vi "COD主界面（列队使用）.vi"() -> (8 "多列列表框":i32(listbox))   [LabVIEW 2016, in "斯坦道CODMn.lvlib"]
uses:
  <vilib>/Utility/miscctls.llb/LVPointTypeDef.ctl
  <vilib>/ptbypt/NI_PtbyPt.lvlib
panel:
  in  "温度补偿":bool
  in  "周期设置":bool
  out "F5":dbl
  out "F4":dbl
  out "F3":dbl
  out "F2":dbl
  out "F1":dbl
  out "F0":dbl
  out "消解压力kPa":dbl format="%#.2f"
  out "权限等级":string
  in  "布尔":bool
  in  "查看曲线":bool
  out "氢氧化钠":dbl
  in  "序列号变更":bool
  out "模块版本号":string
  in  "更新程序":bool
  out "进样无液体告警":bool
  out "60分钟超时报警":bool
  in  "仪器参数":bool
  in  "释放串口":bool
  in  "打开串口":bool
  out "报警数字":i16
  out "CODMn工作状态":T1(ring)
  out "ORP-K":string
  out "ORP-B":string
  out "ORP-A":string
  out "基本量程(显示)":string
  out "测量模式(显示)":string
  out "数据时间":string
  out "断电排液标记":bool
  out "COM":string
  out "空白测试标记":bool
  out "跨度核查标记":bool
  in  "手动控制":bool
  out "启动时间":timestamp format="%<%Y/%m/%d %H:%M:%S>T"
  out "零点核查标记":bool
  out "排液故障":bool
  out "进水样超量程":bool
  out "标样核查标记":bool
  out "平行样测量":bool
  out "加标回收测量":bool
  out "质控样测量":bool
  out "待机":bool
  out "校标错误":bool
  out "校零错误":bool
  out "测量错误":bool
  out "草酸钠报警":bool
  out "高锰酸钾报警":bool
  out "加热故障":bool
  out "温控器故障":bool
  out "ORP故障":bool
  out "排液标记":bool
  out "故障标记":bool
  out "校标标记":bool
  out "校零标记":bool
  out "通讯状态":bool
  out "水样测量":bool
  in  "返回":bool
  in  "校准配置":bool
  out "标度滴定值":dbl
  out "零点滴定值":dbl
  in  "保存":bool
  in  "关闭":bool
  out "仪器时间":timestamp format="%<%Y/%m/%d %H:%M:%S>T"
  out "秒":u16
  out "分":u16
  out "COD浓度（mg/L)":dbl format="%.2g"
  out "进样管":dbl
  out "高锰酸钾":dbl
  out "草酸钠":dbl
  out "硫酸":dbl
  out "实时ORP/光值":dbl
  out "消解温度℃":dbl
  out "加热":bool
  out "搅拌":bool
  out "进硫酸":bool
  out "进加标回收样":bool
  out "进零点核查样":bool
  out "进标液":bool
  out "进蒸馏水":bool
  out "进水样":bool
  out "进草酸钠":bool
  out "进高锰酸钾":bool
  in  "启动":bool
  in  "故障清除":bool
  in  "参数配置":bool
  in  "停止":bool
  in  "单步启动":bool
  out "系统时间":timestamp
  in  "时间校准":bool
  out "模式（受控）":u16
  # "测试时长："
  # "注：遇到加热故障和排液故障时仪器不能正常启动，\n必须排查故障并点击报警清除按钮方可运行。"
  # "mg/L"
  # "校零校标结果"
  # "校零结果："
  # "校零滴定值："
  # "校标结果："
  # "标度滴定值："
  # "零点泵计量值："
  # "标度泵计量值："
  # "校准配置界面"
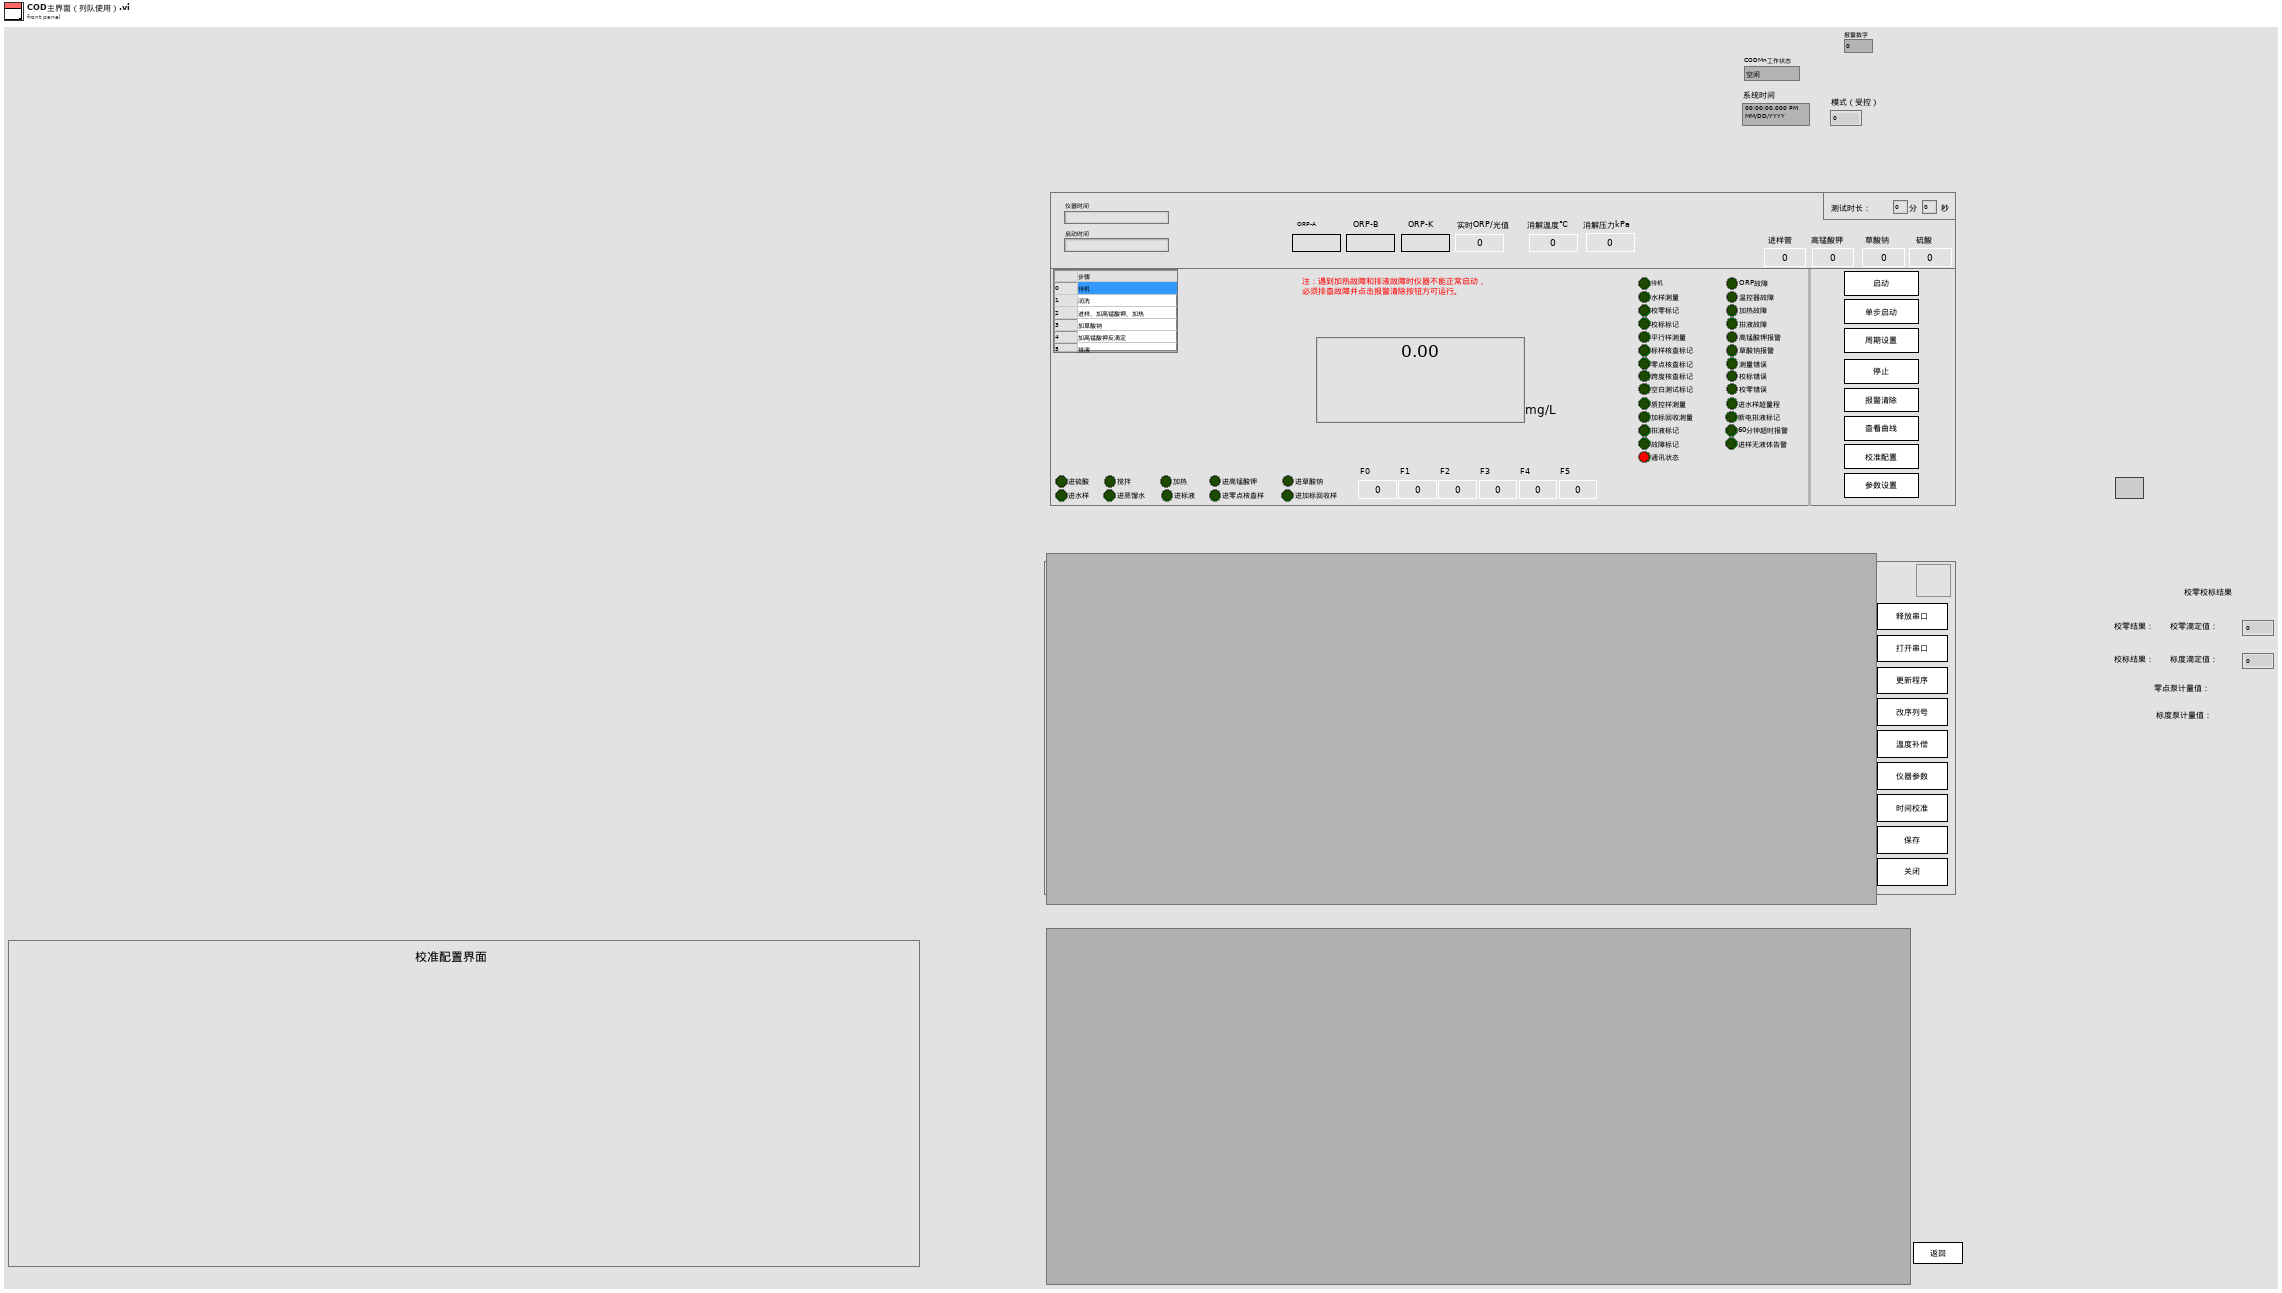
[diagram p1: front panel]
types:
  T1 = enum16{"空闲", "水样测试", "标样核查", "零点核查", "跨度核查", "空白测试", "平行样测试", "质控样", "空白校准", "标样校准", "加标回收"}
  T2 = typedef "LVPointTypeDef.ctl" = cluster{"Horizontal":i16, "Vertical":i16}
  T3 = cluster{"Major":u16, "Minor":u16, "Fix":u16, "Build":u16}
  T4 = cluster{"运行模式":enum16{"维护模式", "常规模式", "应急模式", "质控模式"}, "质控频次":enum16{"关闭", "每天", "星期一", "星期二", "星期三", "星期四", "星期五", "星期六", "星期日"}, "空白核查时间":u16, "跨度核查时间":u16, "测量间隔":u16}
  T5 = cluster{"测量量程":dbl, "测量精度":dbl, "测量间隔":dbl, "消解温度":dbl, "消解时长":dbl, "空白校准时间":timestamp, "曲线截距":dbl, "曲线斜率":dbl, "测量检出限":dbl, "测量信号值":dbl, "线性相关系数":dbl, "二次多项式系数":dbl, "标样校准时间":timestamp, "稀释倍数":dbl, "三项式系数":dbl, "空白标定系数":dbl, "量程系数":dbl, "F0/ORPA":dbl, "F1/ORPB":dbl, "F2/ORPK":dbl, "F3":dbl, "F4":dbl, "F5":dbl, "F6":dbl, "F7":dbl, "X0/滴定数":dbl, "量程":dbl}
  T6 = typedef "TimingControl.lvlib/TimingControl.lvclass/国标控制命令.ctl" = enum16{"启动测量", "标样核查", "零点核查", "跨度核查", "空白测试", "平行样测试", "加标回收", "空白校准", "标样校准", "初始化（清洗）", "停止测试", "仪器重启", "校时", "模式设置", "测量间隔设置"}
  T7 = typedef "TimingControl.lvlib/TimingControl.lvclass/测量参数.ctl" = u16
  T8 = enum32{"Bad", "Idle", "Run top level", "Running"}
  T9 = enum8{"Enabled", "Disabled", "Disabled and Grayed Out"}
  T10 = cluster{"因子编码":u32, "单位":u16, "标样参考值":sgl, "水样数据时间":timestamp, "水样实测值":sgl, "水样数据标识":string, "标样数据时间":timestamp, "标样实测值":sgl, "标样数据标识":string, "空白数据时间":timestamp, "空白实测值":sgl, "空白数据标识":string, "零点核查数据时间":timestamp, "零点核查实测值":sgl, "零点核查数据标识":string, "跨度核查数据时间":timestamp, "跨度核查实测值":sgl, "跨度核查数据标识":string, "加标回收数据时间":timestamp, "加标回收实测值":sgl, "加标回收数据标识":string, "平行样数据时间":timestamp, "平行样实测值":sgl, "平行样数据标识":string}
  T11 = cluster{"时间":timestamp, "测量模式":string, "数据类型":string, "检测值":sgl, "单位":string, "数据标识":string, "因子编码":string, "标样参考值":sgl, "ORP-A":sgl, "ORP-B":sgl, "ORP-K":sgl, "COD滴定值":sgl, "高锰酸钾滴定数":sgl, "温度":sgl, "量程":sgl, "LastTime":timestamp, "序列号:":string, "跨度值":sgl, "高锰酸钾原始滴定数":sgl, "F0":sgl, "F1":sgl, "F2":sgl, "F3":sgl, "F4":sgl, "F5":sgl, "启动温度":sgl}
  T12 = cluster{"ORP故障":bool, "温控器故障":bool, "加热故障":bool, "高锰酸钾报警":bool, "草酸钠报警":bool, "测量错误":bool, "校零错误":bool, "校标错误":bool, " 进水样超量程":bool, "排液阀故障":bool, "60分钟超时报警":bool, "进样无液体报警":bool}
  T13 = cluster{"时间":timestamp, "水样计量数":u16, "蒸馏水计量数":u16, "标液计量数":u16, "零点核查计量数":u16, "加标回收计量数":u16, "硫酸计量数":u16, "高锰酸钾计量数":u16, "草酸钠计量数":u16, "更换泵管":string}
  T14 = cluster{"确定":bool, "测量量程":dbl, "测量精度":dbl, "测量间隔":dbl, "消解温度":dbl, "消解时长":dbl, "空白校准时间":timestamp, "曲线截距":dbl, "曲线斜率":dbl, "测量检出限":dbl, "测量信号值":dbl, "线性相关系数":dbl, "二次多项式系数":dbl, "标样校准时间":timestamp, "稀释倍数":dbl, "三项式系数":dbl, "空白标定系数":dbl, "量程系数":dbl, "F0/ORPA":dbl, "F1/ORPB":dbl, "F2/ORPK":dbl, "F3":dbl, "F4":dbl, "F5":dbl, "F6":dbl, "F7":dbl, "X0/滴定数":dbl, "量程":dbl}
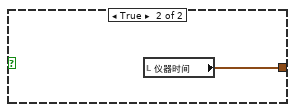
[diagram p6: hidden frame]
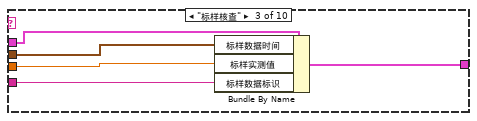
[diagram p12: hidden frame]
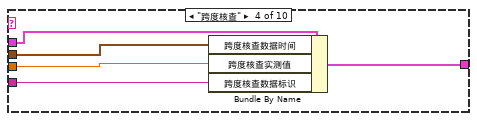
[diagram p13: hidden frame]
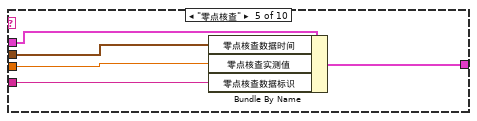
[diagram p14: hidden frame]
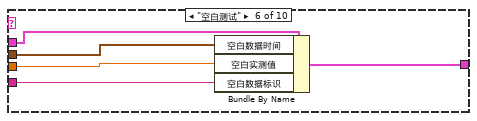
[diagram p15: hidden frame]
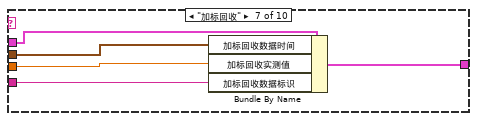
[diagram p16: hidden frame]
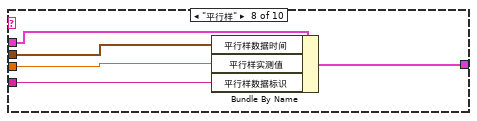
[diagram p17: hidden frame]
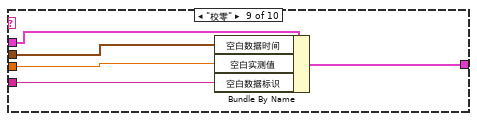
[diagram p18: hidden frame]
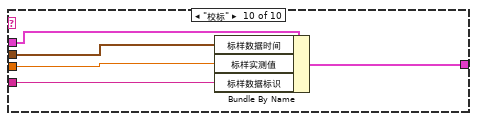
[diagram p19: hidden frame]
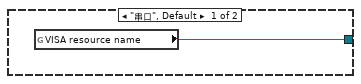
[diagram p20: hidden frame]
diagram:
  n1 = control-ref of="周期设置"() -> (w5:refnum<vi>)
  n2 = call "New TimingControl.vi"("Reference"=w5) -> ("error out"=w3:errorcluster, "TimingControl out"=w4:refnum<class "TimingControl.lvclass">)  [unwired: 9 in]
  n3 = call "taskqueue ref.vi"() -> ("队列输出"=w16:refnum<queue>)  [unwired: 10 in, 1 out]
  n4 = call "task.vi"() -> ()  [unwired: 12 in]
  n5 = flat-sequence {
    tunnel: [errorcluster {"status"=FALSE, "code"=0, "source"=""} ("错误输出")] -> w17
    frame #0 {
      n6 = global write "COD内部交互全局.vi" "量程切换次数"(u8 0 ("量程切换次数")) -> ()
      n7 = global write "COD内部交互全局.vi" "切换量程连续测两次"(FALSE ("切换量程连续测两次")) -> ()
      n8 = property on="窗格" class="Pane"("Origin"=T2 {"Horizontal"=0, "Vertical"=0} ("原点")) -> ()  [unwired: 2 in, 2 out]
      n9 = control-ref of="本VI"() -> (w36:refnum<vi>)
      n10 = property class="VI"(reference=w36) -> ("Library.Version"=w35:T3)  [unwired: 1 in, 2 out]
      n11 = Unbundle By Name(w35) -> ("Major"=w33:u16, "Minor"=w32:u16, "Fix"=w31:u16, "Build"=w30:u16)
      n12 = Format Into String(format string="模块版本号：%d.%d.%d.%d" ("格式字符串"), w33, w32, w31, w30) -> (resulting string=→"模块版本号":string)  [unwired: 2 in, 1 out]
    }
  }
  n13 = while {
    stop <- FALSE stop-if-true
    # "相差60秒自动校时"
    n14 = global read "运行时序全局变量.vi" "多列列表框"() -> (w44:i32)
    n15 = local read "消解温度℃"() -> (w41:dbl)
    n16 = local read "仪器时间"() -> (w51:timestamp)
    n17 = local read "系统时间"() -> (w52:timestamp)
    n18 = Wait (ms)(milliseconds to wait=u32 1000 ("等待时间（毫秒）")) -> ()  [unwired: 1 out]
    n19 = call "消解压力计算.vi"("当前消解温度"=w41) -> ("消解压力"=→"消解压力kPa":dbl)  [unwired: 10 in]
    n20 = Build Array(w51) -> (w50:timestamp[])
    n21 = Build Array(w52) -> (w69:timestamp[])
    n22 = Equal?(x=w44, y=u16 5) -> (x = y?=w46:bool)
    n23 = call <vilib>:"Boolean Crossing PtByPt.vi"("direction"=enum16{"either", "false-true", "true-false"}."false-true", "input"=w46) -> ("crossing"=w43:bool)  [unwired: 1 in]
    n24 = call "DateToHex.vi"("DATE"=w50) -> ("数组"=w63:u16[])  [unwired: 10 in]
    n25 = call "DateToHex.vi"("DATE"=w69) -> ("数组"=w68:u16[])  [unwired: 10 in]
    n26 = case shown="真" w43 {
      frame False {
      }
      frame True {
        # "校准结束后自动更新曲线泵滴定数"
        n27 = global read "CODMN外部API.vi" "远程反控校准CODMn"() -> (w70:bool)
        n28 = case shown="真" w70 {
          frame False {
          }
          frame True {
            # "校准完自动写入公式"
            n29 = global write "CODMN外部API.vi" "远程反控校准CODMn"(FALSE ("远程反控校准CODMn")) -> ()
          }
        }
      }
    }
    n30 = Index Array(array=w63, index=2 ("索引")) -> (element=w65:u16)
    n31 = Index Array(array=w68, index=2 ("索引")) -> (element=w66:u16)
    n32 = Split Number(x=w65) -> (hi(x)=w59:u8)  [unwired: 1 out]
    n33 = Split Number(x=w66) -> (hi(x)=w62:u8)  [unwired: 1 out]
    n34 = To Byte Integer(number=w59) -> (8bit integer=w58:i8)
    n35 = To Byte Integer(number=w62) -> (8bit integer=w61:i8)
    n36 = Subtract(x=w58, y=w61) -> (x-y=w60:i8)
    n37 = Absolute Value(x=w60) -> (abs(x)=w57:i8)
    n38 = local read "通讯状态"() -> (w54:bool)
    n39 = Greater Or Equal?(x=w57, y=i8 5) -> (x >= y?=w55:bool)
    n40 = And(x=w55, y=w54) -> (x .and. y?=w53:bool)
    n41 = case shown="真" w53 {
      frame False {
      }
      frame True {
        # "相差60秒时间自动校准"
        n42 = flat-sequence {
          frame #0 {
            n43 = property on="时间校准" class="Bool (严格)"("Val(Sgnl)"=TRUE ("值(信号)")) -> ()  [unwired: 2 in, 2 out]
          }
          frame #1 {
            n44 = Wait (ms)(milliseconds to wait=u32 500 ("等待时间（毫秒）")) -> ()  [unwired: 1 out]
          }
          frame #2 {
            n45 = property on="时间校准" class="Bool (严格)"("Val(Sgnl)"=FALSE ("值(信号)")) -> ()  [unwired: 2 in, 2 out]
          }
        }
      }
    }
  }
  n46 = while {
    tunnel: w16 -> [w93]
    shift-right: [w85] -> _
    shift-left: 0 -> [w84]
    shift-right: [w76] -> w2
    shift-left: w4 -> [w81]
    shift-right: [w75] -> w1
    shift-left: w3 -> [w80]
    stop <- FALSE stop-if-true
    n47 = global read "CODMn断电保存全局变量.vi" "运行周期"() -> (w95:T4)
    n48 = local read "通讯状态"() -> (w98:bool)
    n49 = Quotient & Remainder(x=w84, y=30) -> (x-y*floor(x/y)=w82:i32)  [unwired: 1 out]
    n50 = Equal To 0?(x=w82) -> (x = 0?=w89:bool)
    n51 = global read "CODMn断电保存全局变量.vi" "CODMn仪器参数"() -> (w97:T5)
    n52 = Unbundle By Name(w95) -> ("测量间隔"=w94:u16)
    n53 = case shown="假" w98 {
      tunnel: [w109 w110] -> w78
      frame False {
        n54 = Get Date/Time In Seconds() -> (seconds since 1Jan1904=w109:timestamp)
      }
      frame True {
        n55 = local read "仪器时间"() -> (w110:timestamp)
      }
    }
    n56 = Bundle By Name(cluster=w97, "测量间隔"=w94) -> (w96:T5)
    n57 = global read "COD测量模式全局.vi" "CODMn工作状态"() -> (w90:T1)
    n58 = Not Equal?(x=w90, y=T1."空闲") -> (x != y?=w77:bool)
    n59 = global write "CODMn断电保存全局变量.vi" "CODMn仪器参数"(w96) -> ()
    n60 = property class="TimingControl"(reference=w81, error in=w80, "Properties:仪器时间"=w78, "Properties:仪器运行状态"=w77) -> (reference out=w76:refnum<class "TimingControl.lvclass">, error out=w75:errorcluster, "Properties:命令输出"=w79:cluster{"启动":bool, "控制命令":T6, "测量参数":T7})
    n61 = Increment(x=w84) -> (x+1=w87:i32)
    n62 = Unbundle By Name(w79) -> ("启动"=w88:bool, "控制命令"=w92:T6)
    n63 = And(x=w88, y=w89) -> (x .and. y?=w91:bool)
    n64 = Select(t=w87, s=w88, f=0) -> (s? t:f=w85:i32)
    n65 = case shown="真" w91 {
      tunnel: w93 -> [_ w106]
      tunnel: w92 -> [_ w105]
      frame False {
      }
      frame True {
        n66 = Get Queue Status(queue=w106) -> (queue out=w104:refnum<queue>, # elements in queue=w103:i32)  [unwired: 2 in, 6 out]
        n67 = Equal To 0?(x=w103) -> (x = 0?=w102:bool)
        n68 = case shown="真" w102 {
          tunnel: w105 -> [_ w108]
          tunnel: w104 -> [_ w107]
          frame False {
          }
          frame True {
            n69 = Enqueue Element(queue=w107, element=w108) -> ()  [unwired: 2 in, 3 out]
          }
        }
      }
    }
    n70 = Wait (ms)(milliseconds to wait=u32 500 ("等待时间（毫秒）")) -> ()  [unwired: 1 out]
  }
  n71 = vi-ref "斯坦道CODMn.lvlib:参数设置页.vi"() -> (w7:refnum<vi>)
  n72 = vi-ref "校准设置页.vi"() -> (w14:refnum<vi>)
  n73 = property class="VI"(reference=w7) -> (reference out=w9:refnum<vi>, "Exec.State"=w8:T8)  [unwired: 1 in, 1 out]
  n74 = property class="VI"(reference=w14) -> (reference out=w12:refnum<vi>, "Exec.State"=w13:T8)  [unwired: 1 in, 1 out]
  n75 = case shown="\"Idle\"" w8 {
    tunnel: w9 -> [w111 w115]
    tunnel: [w111 w112] -> w6
    frame "Bad", Default {
    }
    frame "Idle" {
      n76 = invoke class="VI" method="Run VI"(reference=w115, "Wait until done"=FALSE ("结束前等待"), "Auto Dispose Ref"=TRUE ("自动销毁引用")) -> (reference out=w112:refnum<vi>)  [unwired: 2 in, 4 out]
    }
  }
  n77 = case shown="\"Idle\"" w13 {
    tunnel: w12 -> [w116 w120]
    tunnel: [w116 w117] -> w11
    frame "Bad", Default {
    }
    frame "Idle" {
      n78 = invoke class="VI" method="Run VI"(reference=w120, "Wait until done"=FALSE ("结束前等待"), "Auto Dispose Ref"=TRUE ("自动销毁引用")) -> (reference out=w117:refnum<vi>)  [unwired: 2 in, 4 out]
    }
  }
  n79 = call "Close TimingControl.vi"("error in (no error)"=w1, "TimingControl in"=w2) -> ()  [unwired: 9 in, 1 out]
  n80 = Obtain Queue(name (unnamed)="CODMn", element data type=cluster{"命令":string} {"命令"="启用模块"} ("元素")) -> (queue out=w27:refnum<queue>, error out=w26:errorcluster)  [unwired: 3 in, 1 out]
  n81 = while {
    stop <- FALSE stop-if-true
    # "赋值循环"
    n82 = flat-sequence {
      frame #0 {
        # "局部变量给内部交互用全局变量"
        n83 = local read "待机"() -> (w128:bool)
        n84 = local read "实时ORP/光值"() -> (w123:dbl)
        n85 = local read "消解温度℃"() -> (w124:dbl)
        n86 = local read "多列列表框"() -> (w130:i32)
        n87 = local read "故障标记"() -> (w131:bool)
        n88 = local read "高锰酸钾"() -> (w125:dbl)
        n89 = global write "COD内部交互全局.vi" "待机"(w128) -> ()
        n90 = local read "COD浓度（mg/L)"() -> (w129:dbl)
        n91 = local read "CODMn工作状态"() -> (w132:T1)
        n92 = local read "断电排液标记"() -> (w126:bool)
        n93 = local read "高锰酸钾报警"() -> (w127:bool)
        n94 = global write "COD内部交互全局.vi" "故障标记"(w131) -> ()
        n95 = global write "COD内部交互全局.vi" "ORP显示"(w123) -> ()
        n96 = global write "COD内部交互全局.vi" "高锰酸钾"(w125) -> ()
        n97 = global write "COD内部交互全局.vi" "实时温度"(w124) -> ()
        n98 = global write "运行时序全局变量.vi" "多列列表框"(w130) -> ()
        n99 = global write "COD浓度全局变量.vi" "COD浓度（mg/L)"(w129) -> ()
        n100 = global write "COD内部交互全局.vi" "断电排液标记"(w126) -> ()
        n101 = global write "COD内部交互全局.vi" "高锰酸钾报警"(w127) -> ()
        n102 = global write "COD测量模式全局.vi" "CODMn工作状态"(w132) -> ()
      }
    }
    n103 = flat-sequence {
      frame #0 {
        # "断电保存全局给局部变量"
        n104 = global read "CODMn断电保存全局变量.vi" "启动时间"() -> (→"启动时间":timestamp)
      }
    }
    n105 = flat-sequence {
      frame #0 {
        # "显示量程说明"
        n106 = global read "COD内部交互全局.vi" "通讯状态"() -> (→"通讯状态":bool)
        n107 = global read "CODMn断电保存全局变量.vi" "MB通信方式选择"() -> (w198:enum16{"串口", "TCP"})
        n108 = case shown="\"TCP\"" w198 {
          tunnel: [w201 w202] -> w200
          frame "串口", Default {
            n109 = global read "CODMn断电保存全局变量.vi" "VISA resource name"() -> (w201:refnum<visa-resource-name>)
          }
          frame "TCP" {
            n110 = global read "CODMn断电保存全局变量.vi" "IP"() -> (w202:string)
          }
        }
        "COM" <- w200
      }
    }
    n111 = flat-sequence {
      frame #0 {
        # "权限隐藏和显示功能"
        n112 = global read "CODMN外部API.vi" "权限等级"() -> (w208:enum16{"一级权限", "二级权限", "三级权限", "超级权限"})
        n113 = global read "CODMn断电保存全局变量.vi" "常规版/认证版"() -> (w204:enum16{"常规版-酸性", "常规版-碱性", "认证版", "浮台版"})
        n114 = case shown="\"二级权限\"" w208 {
          tunnel: [w213 FALSE w218 w220] -> w205
          tunnel: ["一级权限" "二级权限" "三级权限" "超级权限"] -> w207
          tunnel: [w213 TRUE w218 w220] -> w206
          frame "一级权限", Default {
            w213 = FALSE
          }
          frame "二级权限" {
          }
          frame "三级权限" {
            w218 = TRUE
          }
          frame "超级权限" {
            w220 = TRUE
          }
        }
        "权限等级" <- w207
        n115 = global read "CODMn断电保存全局变量.vi" "CODMn系统周期测试?"() -> (w209:bool)
        n116 = case shown="\"浮台版\"" w204 {
          tunnel: [T9."Enabled" ("禁用") T9."Enabled" ("禁用") T9."Disabled and Grayed Out" ("禁用") T9."Enabled" ("禁用")] -> _
          tunnel: [i32[] [2] ("禁用项[]") i32[] [2] ("禁用项[]") i32[] [] ("禁用项[]") i32[] [2] ("禁用项[]")] -> _
          tunnel: [w231 w236 T9."Disabled and Grayed Out" ("禁用") w247] -> _
          tunnel: [w230 FALSE FALSE TRUE] -> _
          tunnel: [w231 w236 T9."Disabled and Grayed Out" ("禁用") w247] -> w212
          tunnel: [w230 TRUE FALSE FALSE] -> w211
          frame "常规版-酸性", Default {
            w230 = FALSE
            w231 = T9."Enabled" ("禁用")
          }
          frame "常规版-碱性" {
            w236 = T9."Enabled" ("禁用")
          }
          frame "认证版" {
            w242 = u16 1 items=["水样测试"=1, "标样核查"=2, "零点核查"=3, "跨度核查"=4, "空白测试"=5, "平行样"=6, "加标回收"=7] ("测量模式(公式)")
            n117 = global write "CODMn断电保存全局变量.vi" "测量模式(公式)"(w242) -> ()
          }
          frame "浮台版" {
            w247 = T9."Enabled" ("禁用")
          }
        }
        n118 = global read "CODMn断电保存全局变量.vi" "运行周期"() -> (w210:T4)
        n119 = case shown="真" w209 {
          tunnel: w210 -> [_ w225]
          tunnel: [T9."Enabled" ("禁用") w223] -> _
          frame False {
          }
          frame True {
            n120 = Unbundle By Name(w225) -> ("运行模式"=w224:enum16{"维护模式", "常规模式", "应急模式", "质控模式"})
            n121 = case shown="\"维护模式\", 默认" w224 {
              tunnel: [T9."Enabled" ("禁用") T9."Disabled and Grayed Out" ("禁用") T9."Disabled and Grayed Out" ("禁用") T9."Disabled and Grayed Out" ("禁用")] -> w223
              frame "维护模式", Default {
              }
              frame "常规模式" {
              }
              frame "应急模式" {
              }
              frame "质控模式" {
              }
            }
          }
        }
        n122 = property on="更新程序" class="Bool (严格)"("Visible"=w205) -> ()  [unwired: 2 in, 2 out]
        n123 = property on="释放串口" class="Bool"("Visible"=w206) -> ()  [unwired: 2 in, 2 out]
        n124 = property on="打开串口" class="Bool"("Visible"=w206) -> ()  [unwired: 2 in, 2 out]
        n125 = property on="序列号变更" class="Bool"("Visible"=w205) -> ()  [unwired: 2 in, 2 out]
        n126 = property on="氢氧化钠" class="DigNum (严格)"("Visible"=w211) -> ()  [unwired: 2 in, 2 out]
        n127 = control-ref of="进样管"() -> (w203:refnum<vi>)
        n128 = property class="DigNum (严格)"(reference=w203, "DisabledEnum"=w212) -> ()  [unwired: 1 in, 2 out]
      }
    }
    n129 = flat-sequence {
      frame #0 {
        # "测量数据区"
        n130 = global read "CODMn断电保存全局变量.vi" "测量数据区"() -> (w145:T10)
        n131 = global read "COD内部交互全局.vi" "data"() -> (w150:T11)
        n132 = global read "COD测量模式全局.vi" "测量模式文字实时"() -> (w136:string)
        "测量模式(显示)" <- w136
        n133 = global read "CODMn断电保存全局变量.vi" "水样测试量程"() -> (w138:enum16{"L", "H"})
        n134 = Unbundle By Name(w145) -> ("水样实测值"=w142:sgl)
        n135 = global read "CODMn断电保存全局变量.vi" "测量模式"() -> (w134:string)
        n136 = Unbundle By Name(w150) -> ("时间"=w149:timestamp, "检测值"=w148:sgl, "数据标识"=w147:string)
        n137 = feedback-in #1(w145) -> ()
        n138 = feedback #1(w145) -> (w144:T10)
        n139 = Unbundle By Name(w144) -> ("水样实测值"=w143:sgl)
        n140 = case shown="\"水样测试\"" w136 {
          tunnel: w145 -> [w151 w156 w161 w166 w171 w176 w181 w186 w191 w196]
          tunnel: [w151 w155 w160 w162 w170 w175 w180 w185 w187 w195] -> w146
          tunnel: w149 -> [_ w154 w159 w165 w169 w174 w179 w184 w190 w194]
          tunnel: w148 -> [_ w153 w158 w164 w168 w173 w178 w183 w189 w193]
          tunnel: w147 -> [_ w152 w157 w163 w167 w172 w177 w182 w188 w192]
          frame "", Default {
          }
          frame "水样测试" {
            n141 = Bundle By Name(cluster=w156, "水样数据时间"=w154, "水样实测值"=w153, "水样数据标识"=w152) -> (w155:T10)
          }
          frame "标样核查" {
            n142 = Bundle By Name(cluster=w161, "标样数据时间"=w159, "标样实测值"=w158, "标样数据标识"=w157) -> (w160:T10)
          }
          frame "跨度核查" {
            n143 = Bundle By Name(cluster=w166, "跨度核查数据时间"=w165, "跨度核查实测值"=w164, "跨度核查数据标识"=w163) -> (w162:T10)
          }
          frame "零点核查" {
            n144 = Bundle By Name(cluster=w171, "零点核查数据时间"=w169, "零点核查实测值"=w168, "零点核查数据标识"=w167) -> (w170:T10)
          }
          frame "空白测试" {
            n145 = Bundle By Name(cluster=w176, "空白数据时间"=w174, "空白实测值"=w173, "空白数据标识"=w172) -> (w175:T10)
          }
          frame "加标回收" {
            n146 = Bundle By Name(cluster=w181, "加标回收数据时间"=w179, "加标回收实测值"=w178, "加标回收数据标识"=w177) -> (w180:T10)
          }
          frame "平行样" {
            n147 = Bundle By Name(cluster=w186, "平行样数据时间"=w184, "平行样实测值"=w183, "平行样数据标识"=w182) -> (w185:T10)
          }
          frame "校零" {
            n148 = Bundle By Name(cluster=w191, "空白数据时间"=w190, "空白实测值"=w189, "空白数据标识"=w188) -> (w187:T10)
          }
          frame "校标" {
            n149 = Bundle By Name(cluster=w196, "标样数据时间"=w194, "标样实测值"=w193, "标样数据标识"=w192) -> (w195:T10)
          }
        }
        n150 = feedback #2(w138) -> (w139:enum16{"L", "H"})
        n151 = feedback-in #2(w138) -> ()
        n152 = feedback #3(w134) -> (w135:string)
        n153 = feedback-in #3(w134) -> ()
        n154 = Not Equal?(x=w135, y=w134) -> (x != y?=w133:bool)
        n155 = Not Equal?(x=w139, y=w138) -> (x != y?=w137:bool)
        n156 = Not Equal?(x=w142, y=w143) -> (x != y?=w141:bool)
        n157 = Compound Arithmetic op=OR ("复合运算")(w141, w137, w133) -> (w140:bool)
        n158 = case shown="真" w140 {
          frame False {
          }
          frame True {
            # "水样值发送改变存储本地"
            n159 = call "配置文件保存.vi"() -> ()  [unwired: 12 in]
          }
        }
        n160 = global write "CODMn断电保存全局变量.vi" "测量数据区"(w146) -> ()
      }
    }
    n161 = Wait (ms)(milliseconds to wait=u32 1000 ("等待时间（毫秒）")) -> ()  [unwired: 1 out]
  }
  n162 = flat-sequence {
    tunnel: w17 -> [_]
    frame #0 {
      n163 = vi-ref "斯坦道CODMn.lvlib:关键参数交互.vi"() -> (w268:refnum<vi>)
      n164 = vi-ref "斯坦道CODMn.lvlib:时间-温度曲线(子VI).vi"() -> (w259:refnum<vi>)
      n165 = property class="VI"(reference=w268, error in=errorcluster {"status"=FALSE, "code"=0, "source"=""} ("错误输出")) -> ("Name"=w267:string)  [unwired: 2 out]
      n166 = vi-ref "斯坦道CODMn.lvlib:高锰酸钾-ORP滴定曲线(子VI).vi"() -> (w277:refnum<vi>)
      n167 = vi-ref "斯坦道CODMn.lvlib:日志报警状态存储 (子VI).vi"() -> (w290:refnum<vi>)
      n168 = vi-ref "斯坦道CODMn.lvlib:待机状态数据存储写入和切换量程(子VI).vi"() -> (w297:refnum<vi>)
      n169 = property class="VI"(reference=w259, error in=errorcluster {"status"=FALSE, "code"=0, "source"=""} ("错误输出")) -> ("Name"=w258:string)  [unwired: 2 out]
      n170 = property class="VI"(reference=w290, error in=errorcluster {"status"=FALSE, "code"=0, "source"=""} ("错误输出")) -> ("Name"=w289:string)  [unwired: 2 out]
      n171 = property class="VI"(reference=w277, error in=errorcluster {"status"=FALSE, "code"=0, "source"=""} ("错误输出")) -> ("Name"=w278:string)  [unwired: 2 out]
      n172 = Open VI Reference(type specifier VI Refnum (for type only)=refnum<vi> refnum, vi path=w267, options=128 ("选项")) -> (vi reference=w269:refnum<vi>, error out=w265:errorcluster)  [unwired: 3 in]
      n173 = property class="VI"(reference=w297, error in=errorcluster {"status"=FALSE, "code"=0, "source"=""} ("错误输出")) -> ("Name"=w296:string)  [unwired: 2 out]
      n174 = Open VI Reference(type specifier VI Refnum (for type only)=refnum<vi> refnum, vi path=w258, options=128 ("选项")) -> (vi reference=w260:refnum<vi>, error out=w256:errorcluster)  [unwired: 3 in]
      n175 = Open VI Reference(type specifier VI Refnum (for type only)=refnum<vi> refnum, vi path=w289, options=128 ("选项")) -> (vi reference=w273:refnum<vi>, error out=w287:errorcluster)  [unwired: 3 in]
      n176 = Open VI Reference(type specifier VI Refnum (for type only)=refnum<vi> refnum, vi path=w278, options=128 ("选项")) -> (vi reference=w276:refnum<vi>, error out=w280:errorcluster)  [unwired: 3 in]
      n177 = call-by-ref "?"(reference=w260, error in=w256) -> (reference out=w254:refnum<vi>, error out=w255:errorcluster)  [unwired: 12 in]
      n178 = call-by-ref "?"(reference=w269, error in=w265, "量程选择"=enum16{"低量程", "高量程"}."低量程", "模型"=enum32{"线性", "多项式", "折线"}."线性") -> (reference out=w263:refnum<vi>, error out=w264:errorcluster)  [unwired: 10 in]
      n179 = Close Reference(reference=w254, error in (no error)=w255) -> ()  [unwired: 1 out]
      n180 = Close Reference(reference=w263, error in (no error)=w264) -> ()  [unwired: 1 out]
      n181 = call-by-ref "?"(reference=w273, error in=w287) -> (reference out=w285:refnum<vi>, error out=w286:errorcluster)  [unwired: 12 in]
      n182 = call-by-ref "?"(reference=w276, error in=w280) -> (reference out=w282:refnum<vi>, error out=w281:errorcluster)  [unwired: 12 in]
      n183 = Open VI Reference(type specifier VI Refnum (for type only)=refnum<vi> refnum, vi path=w296, options=128 ("选项")) -> (vi reference=w271:refnum<vi>, error out=w294:errorcluster)  [unwired: 3 in]
      n184 = Close Reference(reference=w285, error in (no error)=w286) -> ()  [unwired: 1 out]
      n185 = Close Reference(reference=w282, error in (no error)=w281) -> ()  [unwired: 1 out]
      n186 = call-by-ref "?"(reference=w271, error in=w294) -> (reference out=w292:refnum<vi>, error out=w293:errorcluster)  [unwired: 12 in]
      n187 = Close Reference(reference=w292, error in (no error)=w293) -> ()  [unwired: 1 out]
    }
  }
  n188 = vi-ref "CODMn通讯.vi"() -> (w18:refnum<vi>)
  n189 = while {
    tunnel: w27 -> [w307]
    tunnel: w26 -> [w306]
    stop <- FALSE stop-if-true
    # "主循环界面显示"
    n190 = flat-sequence {
      frame #0 {
        # "A，B，K"
        # "CODMn读取状态"
        n191 = global read "COD内部交互全局.vi" "ORP、时间"() -> (w454:u16[])
        n192 = To Word Integer(number=w454) -> (16bit integer=w472:i16[])
        n193 = Split 1D Array(array=w472, index=3 ("索引")) -> (first subarray=w456:i16[], second subarray=w471:i16[])
        n194 = global read "CODMn断电保存全局变量.vi" "屏蔽负值"() -> (w452:bool)
        n195 = Index Array(array=w456) -> (element #1=w460:i16, element #2=w459:i16, element #3=w458:i16)  [unwired: 3 in]
        n196 = Index Array(array=w471) -> (element #1=w451:i16, element #2=w470:i16, element #3=w469:i16, element #4=w468:i16)  [unwired: 4 in]
        n197 = case shown="真" w452 {
          selector: w452 -> [w474 _]
          tunnel: w451 -> [w476 w481]
          tunnel: [w475 w484] -> w450
          tunnel: [w474 w480] -> _
          frame False {
            n198 = To Single Precision Float(number=w476) -> (single precision float=w478:sgl)
            n199 = Divide(x=w478, y=sgl 100.0) -> (x/y=w475:sgl)
          }
          frame True {
            n200 = To Single Precision Float(number=w481) -> (single precision float=w482:sgl)
            n201 = Divide(x=w482, y=sgl 100.0) -> (x/y=w479:sgl)
            n202 = Less Or Equal To 0?(x=w479) -> (x <= 0?=w480:bool)
            n203 = case shown="真" w480 {
              tunnel: [w485 sgl 0.015] -> w484
              tunnel: w479 -> [w485 _]
              frame False {
              }
              frame True {
              }
            }
          }
        }
        "COD浓度（mg/L)" <- w450
        n204 = To Single Precision Float(number=w468) -> (single precision float=w462:sgl)
        n205 = Build Array(w460, w459, w458) -> (w457:i16[])
        n206 = To Single Precision Float(number=w470) -> (single precision float=w467:sgl)
        n207 = To Single Precision Float(number=w469) -> (single precision float=w463:sgl)
        n208 = call "HexToDate.vi"("数组"=w457) -> ("DATE"=w461:timestamp[])  [unwired: 10 in]
        n209 = Number To Decimal String(number=w467) -> (decimal integer string=→"ORP-A":string)  [unwired: 1 in]
        n210 = Number To Decimal String(number=w463) -> (decimal integer string=→"ORP-B":string)  [unwired: 1 in]
        n211 = Number To Decimal String(number=w462) -> (decimal integer string=→"ORP-K":string)  [unwired: 1 in]
        n212 = Index Array(array=w461) -> (element=w455:timestamp)  [unwired: 1 in]
        n213 = Format Date/Time String(seconds (now)=w455) -> (date/time string=→"数据时间":string)  [unwired: 2 in]
      }
    }
    n214 = flat-sequence {
      frame #0 {
        # "测量状态显示"
        n215 = global read "COD内部交互全局.vi" "F0-F5"() -> (w358:u16[])
        n216 = global read "COD内部交互全局.vi" "测量状态"() -> (w366:u16[])
        n217 = To Single Precision Float(number=w358) -> (single precision float=w357:sgl[])
        n218 = Index Array(array=w357) -> (element #1=→"F0":sgl, element #2=→"F1":sgl, element #3=→"F2":sgl, element #4=→"F3":sgl, element #5=→"F4":sgl, element #6=→"F5":sgl)  [unwired: 6 in]
        n219 = To Word Integer(number=w366) -> (16bit integer=w376:i16[])
        n220 = Index Array(array=w376, index #1=0 ("索引"), index #4=3 ("索引"), index #14=13 ("索引"), index #15=14 ("索引"), index #21=20 ("索引"), index #32=31 ("索引")) -> (element #1=w380:i16, element #2=w379:i16, element #3=w378:i16, element #4=w362:i16, element #5=→"模式（受控）":i16, element #6=→"进样管":i16, element #7=→"高锰酸钾":i16, element #8=→"草酸钠":i16, element #9=→"硫酸":i16, element #10=w375:i16, element #11=w395:i16, element #12=w371:i16, element #13=→"报警数字":i16, element #14=w401:i16, element #15=w386:i16, element #16=→"多列列表框":i16, element #20=→"氢氧化钠":i16, element #21=w359:i16, element #33=→"分":i16, element #34=→"秒":i16)  [unwired: 28 in, 14 out]
        "CODMn工作状态" <- w362
        n221 = global write "COD内部交互全局.vi" "基本量程实时读取"(w359) -> ()
        n222 = Equal?(x=w362, y=T1."水样测试" ("CODMn工作状态")) -> (x = y?=w360:bool)
        n223 = Build Array(w380, w379, w378) -> (w381:i16[])
        n224 = To Single Precision Float(number=w375) -> (single precision float=→"实时ORP/光值":sgl)
        n225 = Number To Decimal String(number=w359) -> (decimal integer string=→"基本量程(显示)":string)  [unwired: 1 in]
        n226 = Equal?(x=w371, y=u16 1) -> (x = y?=→"排液标记":bool)
        n227 = Equal?(x=w371, y=u16 2) -> (x = y?=→"断电排液标记":bool)
        n228 = Divide(x=w395, y=u16 10) -> (x/y=→"消解温度℃":dbl)
        n229 = Divide(x=w401, y=u16 1000) -> (x/y=→"零点滴定值":dbl)
        n230 = Divide(x=w386, y=u16 1000) -> (x/y=→"标度滴定值":dbl)
        n231 = case shown="真" w360 {
          tunnel: w359 -> [_ w404]
          frame False {
          }
          frame True {
            n232 = global write "CODMn断电保存全局变量.vi" "水样测试量程"(w404) -> ()
          }
        }
        n233 = call "HexToDate.vi"("数组"=w381) -> ("DATE"=w377:timestamp[])  [unwired: 10 in]
        n234 = Index Array(array=w377) -> (element=→"仪器时间":timestamp)  [unwired: 1 in]
      }
    }
    n235 = flat-sequence {
      frame #0 {
        # "报警状态显示"
        n236 = global read "COD内部交互全局.vi" "报警点位"() -> (w419:bool[])
        n237 = Index Array(array=w419, index #1=0 ("索引")) -> (element #1=w416:bool, element #2=w415:bool, element #3=w414:bool, element #4=w413:bool, element #5=w412:bool, element #6=w411:bool, element #7=w410:bool, element #8=w409:bool, element #9=w408:bool, element #11=w407:bool, element #13=w406:bool, element #14=w405:bool)  [unwired: 13 in, 2 out]
        "ORP故障" <- w416
        "温控器故障" <- w415
        "加热故障" <- w408
        "高锰酸钾报警" <- w410
        "草酸钠报警" <- w409
        "测量错误" <- w414
        "校零错误" <- w413
        "校标错误" <- w412
        "进水样超量程" <- w411
        "排液故障" <- w407
        "60分钟超时报警" <- w406
        "进样无液体告警" <- w405
        n238 = Compound Arithmetic op=OR ("复合运算")(w416, w415, w408, w410, w409, w414, w412, w413, w411, w407, w406) -> (→"故障标记":bool)
        n239 = Bundle By Name(cluster=T12 {"ORP故障"=FALSE, "温控器故障"=FALSE, "加热故障"=FALSE, "高锰酸钾报警"=FALSE, "草酸钠报警"=FALSE, "测量错误"=FALSE, "校零错误"=FALSE, "校标错误"=FALSE, " 进水样超量程"=FALSE, "排液阀故障"=FALSE, "60分钟超时报警"=FALSE, "进样无液体报警"=FALSE} ("报警簇"), "ORP故障"=w416, "温控器故障"=w415, "加热故障"=w408, "高锰酸钾报警"=w410, "草酸钠报警"=w409, "测量错误"=w414, "校零错误"=w413, "校标错误"=w412, "进水样超量程"=w411, "排液阀故障"=w407, "60分钟超时报警"=w406, "进样无液体报警"=w405) -> (w417:T12)
        n240 = global write "COD内部交互全局.vi" "报警簇"(w417) -> ()
      }
    }
    n241 = flat-sequence {
      frame #0 {
        # "CODMn读取状态"
        n242 = global read "COD内部交互全局.vi" "温度"() -> (w449:bool[])
        n243 = global read "COD内部交互全局.vi" "M输出点"() -> (w448:bool[])
        n244 = Index Array(array=w449) -> (element=→"加热":bool)  [unwired: 1 in]
        n245 = Index Array(array=w448) -> (element #1=→"搅拌":bool, element #4=→"进水样":bool, element #5=→"进蒸馏水":bool, element #6=→"进标液":bool, element #7=→"进零点核查样":bool, element #8=→"进加标回收样":bool, element #9=→"进高锰酸钾":bool, element #10=→"进草酸钠":bool, element #11=→"进硫酸":bool)  [unwired: 11 in, 2 out]
      }
    }
    n246 = flat-sequence {
      frame #0 {
        # "工作状态显示"
        n247 = local read "CODMn工作状态"() -> (w317:T1)
        n248 = Not Equal To 0?(x=w317) -> (x != 0?=w316:bool)
        n249 = Equal?(x=w317, y=u16 0) -> (x = y?=→"待机":bool)
        n250 = Equal?(x=w317, y=u16 8) -> (x = y?=→"校零标记":bool)
        n251 = Equal?(x=w317, y=u16 1) -> (x = y?=→"水样测量":bool)
        n252 = Equal?(x=w317, y=u16 9) -> (x = y?=→"校标标记":bool)
        n253 = Equal?(x=w317, y=u16 7) -> (x = y?=→"质控样测量":bool)
        n254 = Equal?(x=w317, y=u16 5) -> (x = y?=→"空白测试标记":bool)
        n255 = Equal?(x=w317, y=u16 4) -> (x = y?=→"跨度核查标记":bool)
        n256 = Equal?(x=w317, y=u16 3) -> (x = y?=→"零点核查标记":bool)
        n257 = Equal?(x=w317, y=u16 2) -> (x = y?=→"标样核查标记":bool)
        n258 = Equal?(x=w317, y=u16 6) -> (x = y?=→"平行样测量":bool)
        n259 = Equal?(x=w317, y=u16 10) -> (x = y?=→"加标回收测量":bool)
        n260 = case shown="真" w316 {
          tunnel: w317 -> [_ w341]
          frame False {
          }
          frame True {
            n261 = case shown="\"水样测试\"" w341 {
              tunnel: [_ u16 0 ("y") u16 1 ("y") u16 2 ("y") u16 3 ("y") u16 4 ("y") u16 6 ("y") _ u16 7 ("y") u16 8 ("y") u16 5 ("y")] -> w340
              frame "空闲", Default {
              }
              frame "水样测试" {
              }
              frame "标样核查" {
              }
              frame "零点核查" {
              }
              frame "跨度核查" {
              }
              frame "空白测试" {
              }
              frame "平行样测试" {
              }
              frame "质控样" {
              }
              frame "空白校准" {
              }
              frame "标样校准" {
              }
              frame "加标回收" {
              }
            }
            n262 = global write "COD内部交互全局.vi" "测量模式数字"(w340) -> ()
          }
        }
      }
    }
    n263 = Get Date/Time In Seconds() -> (seconds since 1Jan1904=→"系统时间":timestamp)
    n264 = First Call?() -> (First Call?: T/F=w305:bool)
    n265 = Wait (ms)(milliseconds to wait=u32 1000 ("等待时间（毫秒）")) -> ()  [unwired: 1 out]
    n266 = case shown="真" w305 {
      tunnel: w307 -> [w423 w434]
      tunnel: w306 -> [w422 w433]
      tunnel: [w423 w425] -> w303
      tunnel: [w422 w424] -> w302
      frame False {
      }
      frame True {
        n267 = Bundle By Name(cluster=cluster{"命令":string} {"命令"=""} ("元素"), "命令"="CODMn读取参数" ("名称（未命名）")) -> (w437:cluster{"命令":string})
        n268 = Bundle By Name(cluster=cluster{"命令":string} {"命令"=""} ("元素"), "命令"="CODMn读取公式" ("名称（未命名）")) -> (w428:cluster{"命令":string})
        n269 = Enqueue Element(queue=w434, element=w437, timeout in ms (-1)=1000 ("超时毫秒(-1)"), error in (no error)=w433) -> (queue out=w427:refnum<queue>, error out=w426:errorcluster)  [unwired: 1 out]
        n270 = Enqueue Element(queue=w427, element=w428, timeout in ms (-1)=1000 ("超时毫秒(-1)"), error in (no error)=w426) -> (queue out=w425:refnum<queue>, error out=w424:errorcluster)  [unwired: 1 out]
      }
    }
    n271 = Get Queue Status(queue=w303, error in (no error)=w302) -> (queue out=w299:refnum<queue>, error out=w298:errorcluster, # elements in queue=w301:i32)  [unwired: 1 in, 5 out]
    n272 = Equal To 0?(x=w301) -> (x = 0?=w300:bool)
    n273 = case shown="真" w300 {
      tunnel: w299 -> [_ w311]
      tunnel: w298 -> [_ w310]
      frame False {
      }
      frame True {
        n274 = Bundle By Name(cluster=cluster{"命令":string} {"命令"=""} ("元素"), "命令"="CODMn读取" ("名称（未命名）")) -> (w313:cluster{"命令":string})
        n275 = Enqueue Element(queue=w311, element=w313, timeout in ms (-1)=1000 ("超时毫秒(-1)"), error in (no error)=w310) -> ()  [unwired: 3 out]
      }
    }
  }
  n276 = while {
    tunnel: w27 -> [w490]
    tunnel: w26 -> [w489]
    tunnel: w11 -> [w488]
    tunnel: w6 -> [w487]
    stop <- FALSE stop-if-true
    # "主线事件"
    n277 = event shown="[6] \"保存\": 值改变" {
      selector: _ -> [_ _ _ _ _ _ _ _ _ _ _ _ _ _ _ _ _ _ _ _ _]
      dyn-events: _ -> [_ _ _ _ _ _ _ _ _ _ _ _ _ _ _ _ _ _ _ _ _]
      timeout: _ -> [_ _ _ _ _ _ _ _ _ _ _ _ _ _ _ _ _ _ _ _ _]
      tunnel: w490 -> [_ _ _ _ w568 _ _ w610 _ _ _ _ _ _ _ w665 w672 w694 w738 w755 _]
      tunnel: w489 -> [_ _ _ _ w567 _ _ w609 _ _ _ _ _ _ _ w664 w671 w693 w737 w754 _]
      tunnel: w488 -> [_ _ _ _ _ _ _ w608 _ _ _ _ _ _ _ _ _ _ _ _ _]
      tunnel: w487 -> [_ _ _ _ w566 _ _ _ _ _ _ _ _ _ _ _ _ _ _ _ _]
      event "单步启动": Value Change {
        n278 = event-data() -> ()  [unwired: 1 in, 6 out]
        n279 = call "CODMn手动控制框.vi"() -> ()  [unwired: 12 in]
      }
      event "启动": Mouse Down {
        n280 = event-data() -> ()  [unwired: 1 in, 8 out]
        n281 = global read "COD内部交互全局.vi" "基本量程实时读取"() -> (w494:enum16{"L", "H", "AUTO"})
        n282 = call "启动测量模式选择对话框.vi"("量程选择"=w494) -> ("标样浓度输出"=w492:dbl, "量程选择输出"=w493:enum16{"L", "H", "AUTO"}, "启动选择输出"=w498:u16)  [unwired: 8 in]
        n283 = Not Equal?(x=w498, y=u16 7) -> (x != y?=w496:bool)
        n284 = Not Equal?(x=w498, y=u16 8) -> (x != y?=w495:bool)
        n285 = And(x=w496, y=w495) -> (x .and. y?=w500:bool)
        n286 = case shown="真" w500 {
          tunnel: w498 -> [_ w515]
          tunnel: w493 -> [_ w506]
          tunnel: w492 -> [_ w505]
          frame False {
            n287 = One Button Dialog(message="请到校准配置里面进行校准操作！" ("消息")) -> ()  [unwired: 1 in, 1 out]
          }
          frame True {
            n288 = case shown="1" w515 {
              tunnel: [u16 4608 ("address") u16 4608 ("address") u16 4608 ("address") u16 4608 ("address") u16 4608 ("address") u16 4608 ("address") u16 4608 ("address") u16 4608 ("address") u16 4608 ("address") u16 4608 ("address")] -> w508
              tunnel: [u16 1 ("address") u16 2 ("address") u16 3 ("address") u16 4 ("address") u16 5 ("address") u16 7 ("address") u16 6 ("address") u16 8 ("address") u16 9 ("address") u16 0 ("address")] -> w512
              tunnel: w505 -> [_ w527 _ _ _ _ _ _ _ _]
              frame 0 {
              }
              frame 1 {
                n289 = flat-sequence {
                  tunnel: w527 -> [w530]
                  frame #0 {
                    n290 = global write "CODMn断电保存全局变量.vi" "标样浓度"(w530) -> ()
                  }
                  frame #1 {
                    n291 = call "配置文件保存.vi"() -> ()  [unwired: 12 in]
                  }
                }
              }
              frame 2 {
              }
              frame 3 {
              }
              frame 4 {
              }
              frame 5 {
              }
              frame 6 {
              }
              frame 7 {
              }
              frame 8 {
              }
              frame 9, Default {
              }
            }
            n292 = case shown="\"H\"" w506 {
              tunnel: [w516 w520 errorcluster {"status"=FALSE, "code"=0, "source"=""} ("error out")] -> w504
              frame "L", Default {
                n293 = call "CODMnMB_api.vi"("STEP"=enum16{"open", "read", "write", "close"}."write", "values"=u16[] [0], "starting address"=u16 4276) -> ("error out"=w516:errorcluster)  [unwired: 6 in, 2 out]
              }
              frame "H" {
                n294 = call "CODMnMB_api.vi"("STEP"=enum16{"open", "read", "write", "close"}."write", "values"=u16[] [1], "starting address"=u16 4276) -> ("error out"=w520:errorcluster)  [unwired: 6 in, 2 out]
              }
              frame "AUTO" {
              }
            }
            n295 = Not Equal?(x=w515, y=u16 9) -> (x != y?=w510:bool)
            n296 = global write "CODMN外部API.vi" "手动启动CODMn"(w510) -> ()
            n297 = call "单步测试一键复位.vi"("Error in"=w504) -> ("error out"=w503:errorcluster)  [unwired: 10 in]
            n298 = call <vilib>:"Clear Errors.vi"("error in (no error)"=w503) -> ("error out"=w502:errorcluster)  [unwired: 5 in, 1 out]
            n299 = Insert Into Array(array=u16[] [] ("values"), index=0 ("索引"), new element=w512) -> (w507:u16[])
            n300 = call "CODMnMB_api.vi"("STEP"=enum16{"open", "read", "write", "close"}."write", "Error in"=w502, "values"=w507, "starting address"=w508) -> ()  [unwired: 5 in, 3 out]
          }
        }
      }
      event "停止": Value Change {
        n301 = event-data() -> ()  [unwired: 1 in, 6 out]
        n302 = Two Button Dialog(message="确认是否停止？" ("消息"), 1:"否" ("F按钮名称（“取消”）"), 2:"是" ("T按钮名称（“确定”）")) -> (T button?=w549:bool)
        n303 = case shown="真" w549 {
          frame False {
          }
          frame True {
            n304 = Obtain Notifier(name (unnamed)="CODMn" ("名称（未命名）"), notification data type=FALSE) -> (notifier out=w555:refnum<notifier>, error out=w553:errorcluster)  [unwired: 2 in, 1 out]
            n305 = Send Notification(notification=TRUE ("通知"), notifier=w555, error in (no error)=w553) -> (notifier out=w552:refnum<notifier>, error out=w551:errorcluster)
            n306 = call "CODMnMB_api.vi"("STEP"=enum16{"open", "read", "write", "close"}."write", "values"=u16[] [11], "starting address"=u16 4608) -> ()  [unwired: 6 in, 3 out]
            n307 = Release Notifier(notifier=w552, error in (no error)=w551) -> ()  [unwired: 1 in, 3 out]
          }
        }
      }
      event "手动控制": Value Change {
        n308 = event-data() -> ()  [unwired: 1 in, 6 out]
        n309 = call "数字密码键盘.vi"() -> ("NewNumber"=w561:u32)  [unwired: 1 in]
        n310 = Equal?(x=w561, y=8.0) -> (x = y?=w562:bool)
        n311 = case shown="假" w562 {
          frame False {
            n312 = call "窗口弹出对话框(子VI).vi"("消息"="密码错误") -> ()  [unwired: 10 in, 1 out]
          }
          frame True {
          }
        }
      }
      event "参数配置": Value Change {
        (unwired) u16 20 ("number of holding registers")
        n313 = event-data() -> ()  [unwired: 1 in, 6 out]
        n314 = invoke on="子面板" class="SubPnl" method="Remove VI"() -> (error out=w565:errorcluster)  [unwired: 3 in, 2 out]
        n315 = property on="窗格" class="Pane"("Origin"=T2 {"Horizontal"=0, "Vertical"=650} ("原点")) -> ()  [unwired: 2 in, 2 out]
        n316 = invoke on="子面板" class="SubPnl" method="Insert VI"(error in=w565, "VI Ref"=w566) -> ()  [unwired: 2 in, 4 out]
        n317 = Bundle By Name(cluster=cluster{"命令":string} {"命令"=""} ("元素"), "命令"="CODMn读取参数" ("名称（未命名）")) -> (w569:cluster{"命令":string})
        n318 = Enqueue Element(queue=w568, element=w569, error in (no error)=w567) -> ()  [unwired: 1 in, 3 out]
      }
      event "布尔": Value Change {
        n319 = event-data() -> ("CtlRef"=w573:refnum<vi>, "NewVal"=w574:bool)  [unwired: 1 in, 4 out]
        n320 = case shown="真" w574 {
          tunnel: w573 -> [_ w577]
          frame False {
            n321 = global write "CODMN外部API.vi" "权限等级"(enum16{"一级权限", "二级权限", "三级权限", "超级权限"}."一级权限" ("权限等级")) -> ()
          }
          frame True {
            n322 = property class="Bool (严格)"(reference=w577, "Value"=FALSE ("值")) -> ()  [unwired: 1 in, 2 out]
            n323 = global read "CODMN外部API.vi" "权限密码"() -> (w578:u32[])
            n324 = global read "CODMN外部API.vi" "权限等级"() -> (w580:enum16{"一级权限", "二级权限", "三级权限", "超级权限"})
            n325 = call "密码权限设置.vi"("权限输入"=w580, "权限密码"=w578) -> ("权限输出"=w579:enum16{"一级权限", "二级权限", "三级权限", "超级权限"})  [unwired: 9 in]
            n326 = global write "CODMN外部API.vi" "权限等级"(w579) -> ()
          }
        }
      }
      event "保存": Value Change {
        n327 = event-data() -> ()  [unwired: 1 in, 6 out]
        n328 = local read "通讯状态"() -> (w581:bool)
        n329 = Two Button Dialog(message="确定保存参数，保存参数将会替换原有参数！" ("消息")) -> (T button?=w583:bool)  [unwired: 2 in]
        n330 = case shown="真" w583 {
          tunnel: w581 -> [_ w584]
          frame False {
          }
          frame True {
            n331 = case shown="真" w584 {
              frame False {
                n332 = One Button Dialog(message="保存失败，当前无通讯！" ("消息")) -> ()  [unwired: 1 in, 1 out]
              }
              frame True {
                n333 = global read "COD内部交互全局.vi" "PID参数"() -> (w593:cluster{"P":dbl, "I":dbl, "D":dbl})
                n334 = One Button Dialog(message="参数保存成功！" ("消息")) -> ()  [unwired: 1 in, 1 out]
                n335 = Unbundle(w593) -> ("P"=w592:dbl, "I"=w591:dbl, "D"=w590:dbl)
                n336 = Build Array(w592, w591, w590) -> (w587:dbl[])
                n337 = global read "COD内部交互全局.vi" "保存参数"() -> (w594:dbl[])
                n338 = call "CODMnMB_api.vi"("STEP"=enum16{"open", "read", "write", "close"}."write", "values"=w587, "starting address"=u16 4313) -> ("error out"=w586:errorcluster)  [unwired: 6 in, 2 out]
                n339 = global read "COD内部交互全局.vi" "采水泵参数"() -> (w595:i32[])
                n340 = call "CODMnMB_api.vi"("STEP"=enum16{"open", "read", "write", "close"}."write", "Error in"=w586, "values"=w594, "starting address"=u16 4272) -> ("error out"=w602:errorcluster)  [unwired: 5 in, 2 out]
                n341 = call "CODMnMB_api.vi"("STEP"=enum16{"open", "read", "write", "close"}."write", "Error in"=w602, "values"=w595, "starting address"=u16 5596) -> ("error out"=w599:errorcluster)  [unwired: 5 in, 2 out]
                n342 = global read "COD内部交互全局.vi" "泵校准参数"() -> (w596:T13)
                n343 = call <vilib>:"Clear Errors.vi"("error in (no error)"=w599) -> ("error out"=w597:errorcluster)  [unwired: 5 in, 1 out]
                n344 = call "PLC版CODMn泵校准数据插入.vi"("data"=w596, "错误输入（无错误）"=w597) -> ("错误输出"=w598:errorcluster)  [unwired: 8 in]
                n345 = flat-sequence {
                  tunnel: w598 -> [_]
                  frame #0 {
                    n346 = global write "COD内部交互全局.vi" "更换泵管"(FALSE ("更换泵管")) -> ()
                  }
                }
              }
            }
          }
        }
      }
      event "校准配置": Value Change {
        n347 = event-data() -> ()  [unwired: 1 in, 6 out]
        n348 = invoke on="子面板" class="SubPnl" method="Remove VI"() -> (error out=w607:errorcluster)  [unwired: 3 in, 2 out]
        n349 = property on="窗格" class="Pane"("Origin"=T2 {"Horizontal"=0, "Vertical"=1300} ("原点")) -> ()  [unwired: 2 in, 2 out]
        n350 = invoke on="子面板" class="SubPnl" method="Insert VI"(error in=w607, "VI Ref"=w608) -> ()  [unwired: 2 in, 4 out]
        n351 = Bundle By Name(cluster=cluster{"命令":string} {"命令"=""} ("元素"), "命令"="CODMn读取公式" ("名称（未命名）")) -> (w611:cluster{"命令":string})
        n352 = Enqueue Element(queue=w610, element=w611, error in (no error)=w609) -> ()  [unwired: 1 in, 3 out]
      }
      event "返回": Value Change {
        n353 = event-data() -> ()  [unwired: 1 in, 6 out]
        n354 = property on="窗格" class="Pane"("Origin"=T2 {"Horizontal"=0, "Vertical"=0} ("原点")) -> ()  [unwired: 2 in, 2 out]
      }
      event "关闭": Value Change {
        n355 = event-data() -> ()  [unwired: 1 in, 6 out]
        n356 = property on="窗格" class="Pane"("Origin"=T2 {"Horizontal"=0, "Vertical"=0} ("原点")) -> ()  [unwired: 2 in, 2 out]
      }
      event Application Instance Close {
        n357 = event-data() -> ()  [unwired: 1 in, 4 out]
      }
      event "时间校准": Value Change {
        n358 = event-data() -> ()  [unwired: 1 in, 6 out]
        n359 = Get Date/Time In Seconds() -> (seconds since 1Jan1904=w625:timestamp)
        n360 = Build Array(w625) -> (w624:timestamp[])
        n361 = call "DateToHex.vi"("DATE"=w624) -> ("数组"=w622:u16[])  [unwired: 10 in]
        n362 = Insert Into Array(array=u16[] [1] ("values"), index=1 ("索引"), new element=w622) -> (w618:u16[])
        n363 = call "CODMnMB_api.vi"("STEP"=enum16{"open", "read", "write", "close"}."write", "values"=w618, "starting address"=u16 4612) -> ("error out"=w617:errorcluster)  [unwired: 6 in, 2 out]
        n364 = call <vilib>:"Clear Errors.vi"("error in (no error)"=w617) -> ()  [unwired: 5 in, 2 out]
      }
      event "故障清除": Value Change {
        n365 = event-data() -> ()  [unwired: 1 in, 6 out]
        n366 = call "CODMnMB_api.vi"("STEP"=enum16{"open", "read", "write", "close"}."write", "values"=u16[] [1], "starting address"=u16 4611) -> ()  [unwired: 6 in, 3 out]
      }
      event "仪器参数": Value Change {
        n367 = event-data() -> ()  [unwired: 1 in, 6 out]
        n368 = global read "CODMn断电保存全局变量.vi" "CODMn仪器参数"() -> (w629:T5)
        n369 = call "仪器参数设置.vi"("氨氮仪器参数"=w629) -> ("仪器参数设置输出"=w630:T14)  [unwired: 10 in]
        n370 = Unbundle By Name(w630) -> ("确定"=w631:bool)
        n371 = case shown="真" w631 {
          tunnel: w630 -> [_ w633]
          tunnel: w629 -> [_ w632]
          frame False {
          }
          frame True {
            n372 = flat-sequence {
              tunnel: w633 -> [w652]
              tunnel: w632 -> [w651]
              frame #0 {
                n373 = Unbundle By Name(w652) -> ("测量量程"=w650:dbl, "测量精度"=w649:dbl, "测量间隔"=w635:dbl, "消解温度"=w648:dbl, "消解时长"=w647:dbl, "空白校准时间"=w646:timestamp, "曲线截距"=w645:dbl, "曲线斜率"=w644:dbl, "测量检出限"=w643:dbl, "测量信号值"=w642:dbl, "线性相关系数"=w641:dbl, "二次多项式系数"=w640:dbl, "标样校准时间"=w639:timestamp, "稀释倍数"=w638:dbl)
                n374 = Bundle By Name(cluster=w651, "测量量程"=w650, "测量精度"=w649, "测量间隔"=w635, "消解温度"=w648, "消解时长"=w647, "空白校准时间"=w646, "曲线截距"=w645, "曲线斜率"=w644, "测量检出限"=w643, "测量信号值"=w642, "线性相关系数"=w641, "二次多项式系数"=w640, "标样校准时间"=w639, "稀释倍数"=w638) -> (w637:T5)
                n375 = global read "CODMn断电保存全局变量.vi" "运行周期"() -> (w636:T4)
                n376 = Bundle By Name(cluster=w636, "测量间隔"=w635) -> (w634:T4)
                n377 = global write "CODMn断电保存全局变量.vi" "CODMn仪器参数"(w637) -> ()
                n378 = global write "CODMn断电保存全局变量.vi" "运行周期"(w634) -> ()
              }
              frame #1 {
                n379 = call "配置文件保存.vi"() -> ()  [unwired: 12 in]
                n380 = global write "CODMn断电保存全局变量.vi" "关键参数改变"(TRUE ("校准信息改变")) -> ()
              }
            }
          }
        }
      }
      event "查看曲线": Value Change {
        n381 = event-data() -> ()  [unwired: 1 in, 6 out]
        n382 = vi-ref "斯坦道CODMn.lvlib:读取CODMn数据波形新.vi"() -> (w655:refnum<vi>)
        n383 = property class="VI"(reference=w655) -> ("Name"=w661:string)  [unwired: 1 in, 2 out]
        n384 = Open VI Reference(type specifier VI Refnum (for type only)=refnum<vi> refnum, vi path=w661, options=128 ("选项")) -> (vi reference=w659:refnum<vi>, error out=w658:errorcluster)  [unwired: 3 in]
        n385 = call-by-ref "?"(reference=w659, error in=w658) -> (reference out=w656:refnum<vi>, error out=w657:errorcluster)  [unwired: 12 in]
        n386 = Close Reference(reference=w656, error in (no error)=w657) -> ()  [unwired: 1 out]
      }
      event "释放串口": Value Change {
        n387 = event-data() -> ()  [unwired: 1 in, 6 out]
        n388 = Two Button Dialog(message="确认是否释放串口，释放串口将导致通信失败！" ("消息")) -> (T button?=w662:bool)  [unwired: 2 in]
        n389 = case shown="真" w662 {
          tunnel: w665 -> [_ w667]
          tunnel: w664 -> [_ w666]
          frame False {
          }
          frame True {
            n390 = Bundle By Name(cluster=cluster{"命令":string} {"命令"=""} ("元素"), "命令"="停用模块" ("名称（未命名）")) -> (w668:cluster{"命令":string})
            n391 = Enqueue Element(queue=w667, element=w668, error in (no error)=w666) -> ()  [unwired: 1 in, 3 out]
          }
        }
      }
      event "打开串口": Value Change {
        n392 = event-data() -> ()  [unwired: 1 in, 6 out]
        n393 = flat-sequence {
          tunnel: w672 -> [w680]
          tunnel: w671 -> [w679]
          frame #0 {
            n394 = global read "CODMn断电保存全局变量.vi" "VISA resource name"() -> (w683:refnum<visa-resource-name>)
            n395 = global read "CODMn断电保存全局变量.vi" "MB通信方式选择"() -> (w676:enum16{"串口", "TCP"})
            n396 = global read "CODMn断电保存全局变量.vi" "PORT"() -> (w674:string)
            n397 = global read "CODMn断电保存全局变量.vi" "IP"() -> (w675:string)
            n398 = call "串口配置.vi"("PORT"=w674, "IP"=w675, "MB通信方式选择"=w676, "请选择串口:"=w683) -> ("PORT 2"=w677:string, "IP 2"=w678:string, "确认 2"=w681:bool, "VISA资源名称 2"=w682:refnum<visa-resource-name>, "MB通信方式选择 2"=w673:enum16{"串口", "TCP"})  [unwired: 3 in]
            n399 = case shown="真" w681 {
              tunnel: w682 -> [_ w692]
              tunnel: w680 -> [_ w688]
              tunnel: w679 -> [_ w687]
              tunnel: w678 -> [_ w686]
              tunnel: w677 -> [_ w685]
              tunnel: w673 -> [_ w684]
              frame False {
              }
              frame True {
                n400 = global write "CODMn断电保存全局变量.vi" "IP"(w686) -> ()
                n401 = global write "CODMn断电保存全局变量.vi" "PORT"(w685) -> ()
                n402 = global write "CODMn断电保存全局变量.vi" "VISA resource name"(w692) -> ()
                n403 = global write "CODMn断电保存全局变量.vi" "MB通信方式选择"(w684) -> ()
                n404 = Bundle By Name(cluster=cluster{"命令":string} {"命令"=""} ("元素"), "命令"="启用模块" ("名称（未命名）")) -> (w689:cluster{"命令":string})
                n405 = Enqueue Element(queue=w688, element=w689, error in (no error)=w687) -> ()  [unwired: 1 in, 3 out]
              }
            }
          }
          frame #1 {
            n406 = call "配置文件保存.vi"() -> ()  [unwired: 12 in]
          }
        }
      }
      event "更新程序": Value Change {
        n407 = event-data() -> ("CtlRef"=w695:refnum<vi>, "NewVal"=w696:bool)  [unwired: 1 in, 4 out]
        n408 = case shown="真" w696 {
          tunnel: w695 -> [_ w705]
          tunnel: w694 -> [w698 w704]
          tunnel: w693 -> [w697 w703]
          frame False {
            n409 = Bundle By Name(cluster=cluster{"命令":string} {"命令"=""} ("元素"), "命令"="启用模块" ("名称（未命名）")) -> (w699:cluster{"命令":string})
            n410 = Enqueue Element(queue=w698, element=w699, error in (no error)=w697) -> ()  [unwired: 1 in, 3 out]
          }
          frame True {
            n411 = Two Button Dialog(message="警告，非专业人士请勿进行此操作！！！\n请确认是否继续？" ("消息")) -> (T button?=w707:bool)  [unwired: 2 in]
            n412 = case shown="真" w707 {
              tunnel: w705 -> [w723 _]
              tunnel: w704 -> [_ w731]
              tunnel: w703 -> [_ w730]
              tunnel: [errorcluster {"status"=TRUE, "code"=0, "source"=""} ("error out") w724] -> w702
              frame False {
                n413 = property class="Bool (严格)"(reference=w723, "Value"=FALSE ("释放串口")) -> ()  [unwired: 1 in, 2 out]
              }
              frame True {
                n414 = Bundle By Name(cluster=cluster{"命令":string} {"命令"=""} ("元素"), "命令"="CODMn程序更新" ("名称（未命名）")) -> (w734:cluster{"命令":string})
                n415 = Bundle By Name(cluster=cluster{"命令":string} {"命令"=""} ("元素"), "命令"="停用模块" ("名称（未命名）")) -> (w725:cluster{"命令":string})
                n416 = Enqueue Element(queue=w731, element=w734, error in (no error)=w730) -> (queue out=w729:refnum<queue>, error out=w728:errorcluster)  [unwired: 1 in, 1 out]
                n417 = Enqueue Element(queue=w729, element=w725, error in (no error)=w728) -> (error out=w724:errorcluster)  [unwired: 1 in, 2 out]
              }
            }
            n418 = case shown="无错误" w702 {
              frame No Error {
                n419 = call "文件对话框"("start path"=path "D:/SRC") -> ("selected path"=w710:path, "cancelled"=w708:bool)  [unwired: 11 in, 2 out]
                n420 = case shown="假" w708 {
                  tunnel: w710 -> [w715 _]
                  frame False {
                    n421 = Path To String(path=w715) -> (string=w712:string)
                    n422 = Format Into String(format string="  - \"%s\"" ("格式字符串"), initial string="\"C:\\Program Files\\Fatek\\WinProladder\\WProlad.exe\"" ("command line"), w712) -> (resulting string=w713:string)  [unwired: 1 in, 1 out]
                    n423 = call <vilib>:"System Exec.vi"("command line"=w713) -> ("error out"=w716:errorcluster)  [unwired: 7 in, 3 out]
                    n424 = case shown="错误" w716 {
                      tunnel: w712 -> [_ w719]
                      frame No Error {
                      }
                      frame Error {
                        n425 = Format Into String(format string="  - \"%s\"" ("格式字符串"), initial string="\"C:\\Program Files (x86)\\Fatek\\WinProladder\\WProlad.exe\"" ("command line"), w719) -> (resulting string=w717:string)  [unwired: 1 in, 1 out]
                        n426 = call <vilib>:"System Exec.vi"("command line"=w717) -> ()  [unwired: 7 in, 4 out]
                      }
                    }
                  }
                  frame True {
                  }
                }
              }
              frame Error {
              }
            }
          }
        }
      }
      event "序列号变更": Value Change {
        n427 = event-data() -> ()  [unwired: 1 in, 6 out]
        n428 = global read "COD内部交互全局.vi" "序列号:"() -> (w735:string)
        n429 = call "序列号写入.vi"("序列号:"=w735) -> ("确认 2"=w736:bool, "序列号输出"=w739:string)  [unwired: 9 in]
        n430 = case shown="真" w736 {
          tunnel: w739 -> [_ w745]
          tunnel: w738 -> [_ w741]
          tunnel: w737 -> [_ w740]
          frame False {
          }
          frame True {
            n431 = global write "COD内部交互全局.vi" "序列号:"(w745) -> ()
            n432 = Bundle By Name(cluster=cluster{"命令":string} {"命令"=""} ("元素"), "命令"="CODMn序列号写入" ("名称（未命名）")) -> (w742:cluster{"命令":string})
            n433 = Enqueue Element(queue=w741, element=w742, error in (no error)=w740) -> ()  [unwired: 1 in, 3 out]
          }
        }
      }
      event "温度补偿": Value Change {
        n434 = event-data() -> ()  [unwired: 1 in, 6 out]
        n435 = Bundle By Name(cluster=cluster{"命令":string} {"命令"=""} ("元素"), "命令"="CODMn读取参数" ("名称（未命名）")) -> (w756:cluster{"命令":string})
        n436 = vi-ref "斯坦道CODMn.lvlib:温度补偿.vi"() -> (w747:refnum<vi>)
        n437 = Enqueue Element(queue=w755, element=w756, error in (no error)=w754) -> ()  [unwired: 1 in, 3 out]
        n438 = property class="VI"(reference=w747) -> ("Name"=w753:string)  [unwired: 1 in, 2 out]
        n439 = Open VI Reference(type specifier VI Refnum (for type only)=refnum<vi> refnum, vi path=w753, options=128 ("选项")) -> (vi reference=w751:refnum<vi>, error out=w750:errorcluster)  [unwired: 3 in]
        n440 = call-by-ref "?"(reference=w751, error in=w750) -> (reference out=w748:refnum<vi>, error out=w749:errorcluster)  [unwired: 12 in]
        n441 = Close Reference(reference=w748, error in (no error)=w749) -> ()  [unwired: 1 out]
      }
      event Timeout {
        n442 = event-data() -> ()  [unwired: 1 in, 3 out]
      }
    }
  }
  n443 = property class="VI"(reference=w18, error in=w17) -> ("Name"=w19:string)  [unwired: 2 out]
  n444 = Open VI Reference(type specifier VI Refnum (for type only)=refnum<vi> refnum, vi path=w19, options=128 ("选项")) -> (vi reference=w21:refnum<vi>, error out=w23:errorcluster)  [unwired: 3 in]
  n445 = call-by-ref "?"(reference=w21, error in=w23) -> (reference out=w25:refnum<vi>, error out=w24:errorcluster)  [unwired: 12 in]
  n446 = Close Reference(reference=w25, error in (no error)=w24) -> ()  [unwired: 1 out]
